vi "espectro.vi"() -> ()   [LabVIEW 2016]
uses:
  C:/Users/parra/Documents/moke/thorlabs/Thorlabs.MotionControl.Controls.dll
  thorlabs/Thorlabs.MotionControl.Controls.dll
  C:/Users/parra/Documents/moke/thorlabs/Thorlabs.MotionControl.IntegratedStepperMotorsCLI.dll
  thorlabs/Thorlabs.MotionControl.IntegratedStepperMotorsCLI.dll
panel:
  out "XY Graph":cluster{"X":dbl, "Y":dbl}[](graph)
  in  "paso":dbl
  in  "fin":dbl
  in  "inicio":dbl
  in  "CageRotatorControl":refnum<k24>(container)
  # "analizador"
  # "monocromador"
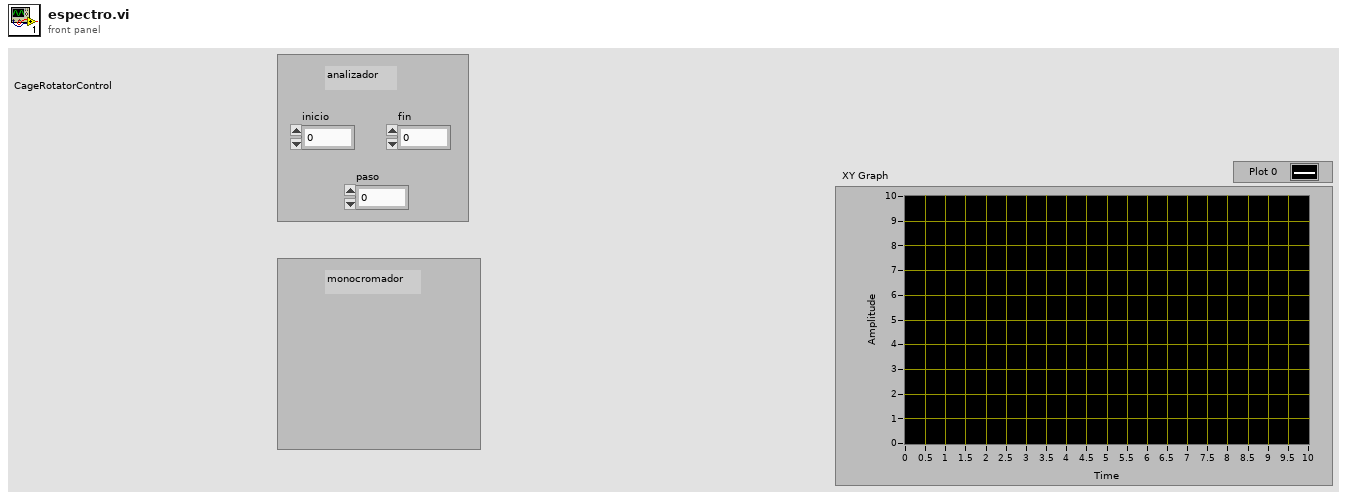
[diagram p1: front panel]
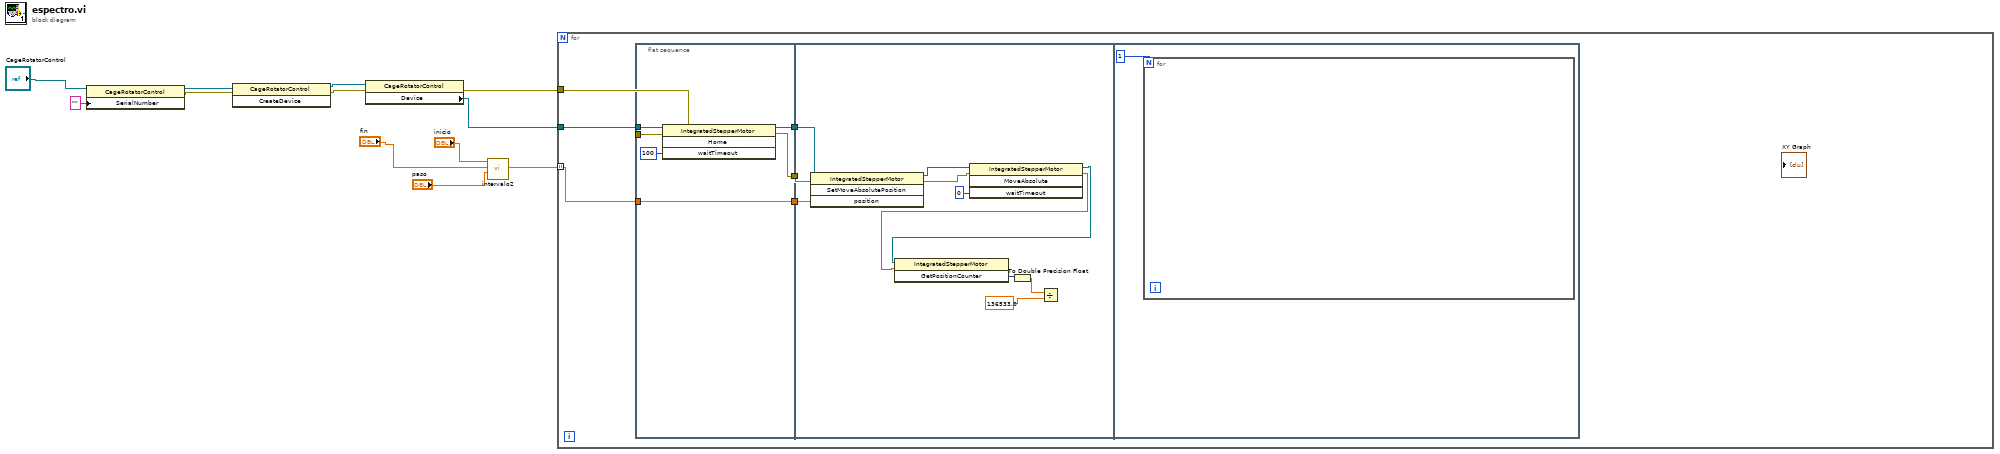
[diagram p0: block diagram]
diagram:
  n1 = property class="CageRotatorControl"(reference="CageRotatorControl", "SerialNumber"="") -> (reference out=w11:refnum<k24>, error out=w6:errorcluster)  [unwired: 1 in]
  n2 = invoke class="CageRotatorControl" method="CreateDevice"(reference=w11, error in=w6) -> (reference out=w8:refnum<k24>, error out=w7:errorcluster)  [unwired: 1 in, 1 out]
  n3 = property class="CageRotatorControl"(reference=w8, error in=w7) -> (error out=w1:errorcluster, "Device"=w2:refnum<k24>)  [unwired: 1 out]
  n4 = call "intervalo2.vi"("incremento"="paso", "fin"="fin", "inicio"="inicio") -> ("Array"=w9:dbl[])  [unwired: 8 in]
  n5 = for {
    tunnel: w9 -> [w14] mode=indexing
    tunnel: w2 -> [w18]
    tunnel: w1 -> [w17]
    n6 = flat-sequence {
      tunnel: w18 -> [w24]
      tunnel: w17 -> [w23]
      tunnel: [w21] -> w16
      tunnel: [w20] -> w15
      tunnel: w14 -> [w19]
      tunnel: [w19] -> w13
      tunnel: w16 -> [w34]
      tunnel: w15 -> [w31]
      tunnel: w13 -> [w30]
      frame #0 {
        n7 = invoke class="IntegratedStepperMotor" method="Home"(reference=w24, error in=w23, "waitTimeout"=100) -> (reference out=w21:refnum<k24>, error out=w20:errorcluster)  [unwired: 1 in, 2 out]
      }
      frame #1 {
        n8 = invoke class="IntegratedStepperMotor" method="SetMoveAbsolutePosition"(reference=w34, error in=w31, "position"=w30) -> (reference out=w32:refnum<k24>, error out=w33:errorcluster)  [unwired: 1 in, 2 out]
        n9 = invoke class="IntegratedStepperMotor" method="MoveAbsolute"(reference=w32, error in=w33, "waitTimeout"=0) -> (reference out=w29:refnum<k24>, error out=w28:errorcluster)  [unwired: 1 in, 2 out]
        n10 = invoke class="IntegratedStepperMotor" method="GetPositionCounter"(reference=w29, error in=w28) -> ("GetPositionCounter"=w27:i32)  [unwired: 1 in, 2 out]
        n11 = To Double Precision Float(number=w27) -> (double precision float=w26:dbl)
        n12 = Divide(x=w26, y=136533.0) -> ()  [unwired: 1 out]
      }
      frame #2 {
        n13 = for {
          N: 1 -> [_]
        }
      }
    }
  }
